vi "JKISM++ Mark As Worker Module.vi"(9 "JKISM Name":string) -> (2 "JKISM Name(marked as worker)":string)   [LabVIEW 2014, in "JKI-State-Machine-Plus.lvlib"]
uses:
  JKI-State-Machine-Plus.lvlib
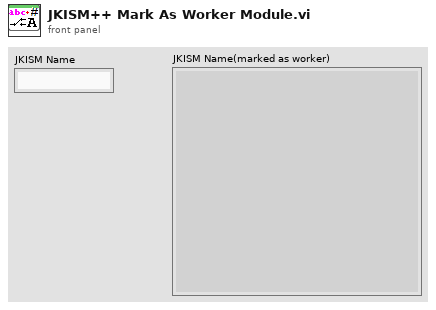
[diagram p1: front panel]
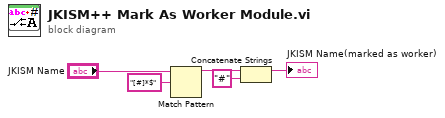
[diagram p0: block diagram]
diagram:
  n1 = Match Pattern(string="JKISM Name", regular expression="[#]*$") -> (before substring=w3:string)  [unwired: 1 in, 3 out]
  n2 = Concatenate Strings(w3, "#" ("string")) -> (→"JKISM Name(marked as worker)":string)
